vi "Find SubVI.vi"(8 "error in":errorcluster, 10 "References":refnum<vi>[](array[refnum]), 11 "Full Vi Name":string) -> (0 "error out":errorcluster)   [LabVIEW 2019, in "Panther Dashboard.lvlib"]
uses:
  Panther Dashboard.lvlib
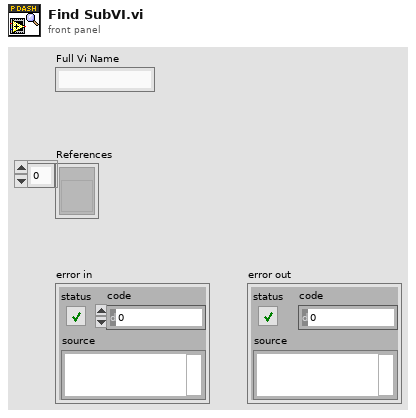
[diagram p1: front panel]
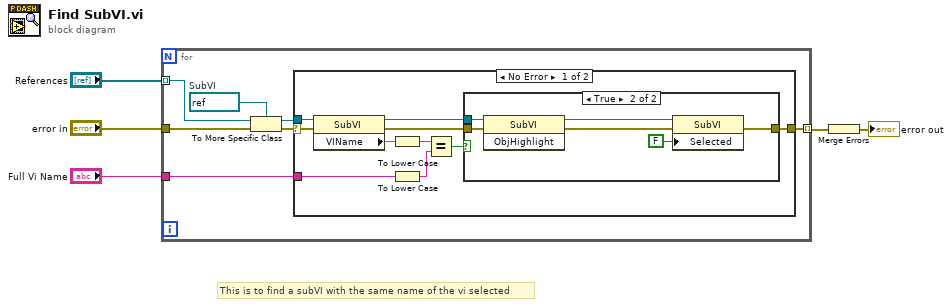
[diagram p0: block diagram]
diagram:
  # "This is to find a subVI with the same name of the vi selected"
  n1 = for {
    tunnel: "References" -> [w9] mode=indexing
    tunnel: "Full Vi Name" -> [w6]
    tunnel: "error in" -> [w11]
    tunnel: [w10] -> w1 mode=indexing
    w8 = refnum<vi> refnum  # SubVI
    n2 = To More Specific Class(target class=w8, reference=w9, error in=w11) -> (specific class reference=w7:refnum<vi>, error out=w12:errorcluster)
    n3 = case shown="No Error" w12 {
      selector: w12 -> [w21 _]
      tunnel: w7 -> [w17 _]
      tunnel: w6 -> [w16 _]
      tunnel: [w20 _] -> w10
      frame No Error {
        n4 = property class="SubVI"(reference=w17, error in=w21) -> (reference out=w15:refnum<vi>, error out=w22:errorcluster, "VIName"=w19:string)
        n5 = To Lower Case(string=w19) -> (all lower case string=w14:string)
        n6 = To Lower Case(string=w16) -> (all lower case string=w13:string)
        n7 = Equal?(x=w14, y=w13) -> (x = y?=w18:bool)
        n8 = case shown="True" w18 {
          tunnel: w15 -> [_ w27]
          tunnel: w22 -> [w23 w29]
          tunnel: [w23 w26] -> w20
          frame False {
          }
          frame True {
            n9 = invoke class="SubVI" method="ObjHighlight"(reference=w27, error in=w29) -> (reference out=w25:refnum<vi>, error out=w28:errorcluster)  [unwired: 1 in, 1 out]
            n10 = property class="SubVI"(reference=w25, error in=w28, "Selected"=FALSE) -> (error out=w26:errorcluster)  [unwired: 1 out]
          }
        }
      }
      frame Error {
      }
    }
  }
  n11 = Merge Errors(w1) -> (→"error out":errorcluster)
